vi "Configure Low Frequency Output.vi"(0 "VISA resource name":refnum<visa-resource-name>, 1 "Enable Low Frequency Output (T:Enable)":bool=TRUE, 5 "Low Frequency Output Amplitude (0 VP)":dbl, 7 "Low Frequency Source (0: Internal1 Monitor)":u16(ring) items=["Internal1 Monitor", "Internal2 Monitor", "Function Generator1", "Function Generator2"], 9 "Waveform Type (0: Sine)":u16(ring) items=["Sine", "Triangle", "Square", "Ramp", "Noise", "Dual-Sine", "Swept-Sine", "DC", "Pulse"], 11 "error in (no error)":errorcluster, 12 "Internal Frequency (400 Hz)":dbl=400.0, 13 "Alternate Internal Frequency (400 Hz)":dbl=400.0) -> (4 "VISA resource name out":refnum<visa-resource-name>, 15 "error out":errorcluster)   [LabVIEW 2014, in "Agilent PSG MXG Series.lvlib"]
doc: "Configures the low frequency output.\n\n<B>Notes:</B>\n(1) This VI is <B>NOT</B> valid in E8247C, N5161A, N5162A, N5181A, N5182A, N5171B, N5172B, N5181B, N5182B.\n\n(2) For E8257D, E8267D, this VI is valid only when the instrument installs <B>Option UNT</B> (AM, FM, phase modulation, and LF output).\n\n(3) Use Configure Modulation (LF Output).vi to configure the low frequency output for N5171B, N5172B, N5181B, N5182B."
uses:
  Agilent PSG MXG Series.lvlib
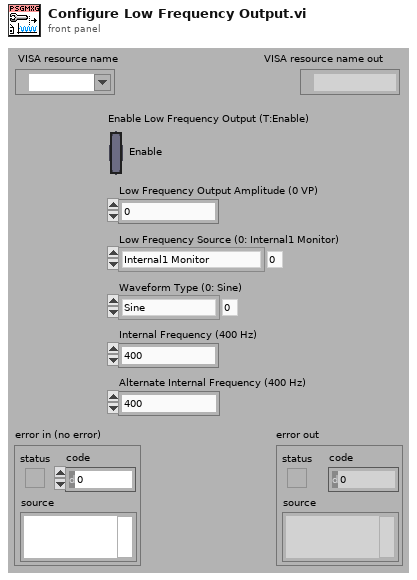
[diagram p1: front panel]
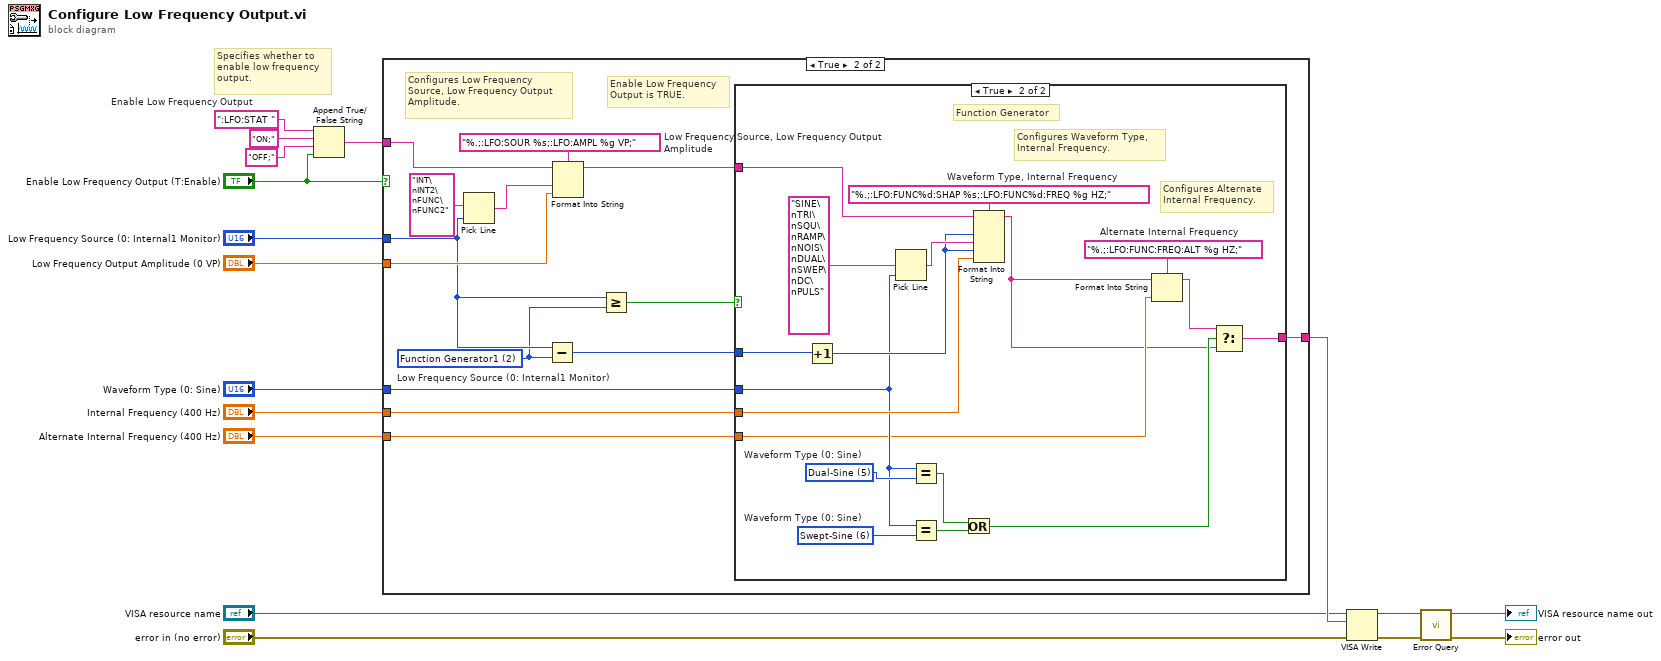
[diagram p0: block diagram]
diagram:
  w17 = ":LFO:STAT "  # Enable Low Frequency Output
  # "Specifies whether to\nenable low frequency\noutput."
  n1 = Append True/False String(1:"Enable Low Frequency Output (T:Enable)", 2:"OFF;" ("false string"), 3:"ON;" ("true string"), 4:w17) -> (0:w13:string)
  n2 = case shown="True" "Enable Low Frequency Output (T:Enable)" {
    tunnel: "Low Frequency Source (0: Internal1 Monitor)" -> [_ w24]
    tunnel: w13 -> [w18 w30]
    tunnel: "Low Frequency Output Amplitude (0 VP)" -> [_ w28]
    tunnel: "Waveform Type (0: Sine)" -> [_ w27]
    tunnel: "Internal Frequency (400 Hz)" -> [_ w26]
    tunnel: [w18 w19] -> w5
    tunnel: "Alternate Internal Frequency (400 Hz)" -> [_ w20]
    frame False {
      # "Enable Low Frequency\nOutput is FALSE."
    }
    frame True {
      w22 = u16 2 items=["Internal1 Monitor", "Internal2 Monitor", "Function Generator1", "Function Generator2"]  # Low Frequency Source (0: Internal1 Monitor)
      w29 = "%.;:LFO:SOUR %s;:LFO:AMPL %g VP;"  # Low Frequency Source, Low Frequency Output Amplitude
      # "Configures Low Frequency\nSource, Low Frequency Output\nAmplitude."
      # "Enable Low Frequency\nOutput is TRUE."
      n3 = Pick Line(multi-line string="INT\nINT2\nFUNC\nFUNC2", line index=w24) -> (output string=w31:string)  [unwired: 1 out]
      n4 = Subtract(x=w24, y=w22) -> (x-y=w23:u16)
      n5 = Format Into String(format string=w29, initial string=w30, w31, w28) -> (resulting string=w25:string)  [unwired: 1 in, 1 out]
      n6 = Greater Or Equal?(x=w24, y=w22) -> (x >= y?=w21:bool)
      n7 = case shown="True" w21 {
        tunnel: w27 -> [_ w42]
        tunnel: w26 -> [_ w48]
        tunnel: w25 -> [w33 w47]
        tunnel: w23 -> [_ w46]
        tunnel: w20 -> [_ w38]
        tunnel: [w33 w34] -> w19
        frame False {
          # "Internal Monitor"
        }
        frame True {
          w39 = "%.;:LFO:FUNC:FREQ:ALT %g HZ;"  # Alternate Internal Frequency
          w43 = u16 6 items=["Sine", "Triangle", "Square", "Ramp", "Noise", "Dual-Sine", "Swept-Sine", "DC", "Pulse"]  # Waveform Type (0: Sine)
          w44 = u16 5 items=["Sine", "Triangle", "Square", "Ramp", "Noise", "Dual-Sine", "Swept-Sine", "DC", "Pulse"]  # Waveform Type (0: Sine)
          w51 = "%.;:LFO:FUNC%d:SHAP %s;:LFO:FUNC%d:FREQ %g HZ;"  # Waveform Type, Internal Frequency
          # "Configures Alternate\nInternal Frequency."
          # "Function Generator"
          # "Configures Waveform Type,\nInternal Frequency."
          n8 = Increment(x=w46) -> (x+1=w45:u16)
          n9 = Pick Line(multi-line string="SINE\nTRI\nSQU\nRAMP\nNOIS\nDUAL\nSWEP\nDC\nPULS", line index=w42) -> (output string=w49:string)  [unwired: 1 out]
          n10 = Equal?(x=w42, y=w44) -> (x = y?=w41:bool)
          n11 = Equal?(x=w42, y=w43) -> (x = y?=w40:bool)
          n12 = Or(x=w41, y=w40) -> (x .or. y?=w37:bool)
          n13 = Format Into String(format string=w51, initial string=w47, w45, w49, w45, w48) -> (resulting string=w35:string)  [unwired: 1 in, 1 out]
          n14 = Format Into String(format string=w39, initial string=w35, w38) -> (resulting string=w36:string)  [unwired: 1 in, 1 out]
          n15 = Select(t=w36, s=w37, f=w35) -> (s? t:f=w34:string)
        }
      }
    }
  }
  n16 = VISA Write(VISA resource name="VISA resource name", write buffer=w5, error in (no error)="error in (no error)") -> (VISA resource name out=w11:refnum<visa-resource-name>, error out=w10:errorcluster)  [unwired: 1 out]
  n17 = call "Error Query.vi"("error in (no error)"=w10, "VISA resource name"=w11) -> ("error out"=→"error out":errorcluster, "VISA resource name out"=→"VISA resource name out":refnum<visa-resource-name>)  [unwired: 8 out]
